vi "SetAttributeViBoolean.vi"(7 "AttributeValue (Off)":bool, 8 "error in (no error)":errorcluster {"code" format="%.0x"}, 9 "AttributeID":u32(ring)=1150179 items=["ACQUISITION_ADC_DITHER_AUTO_ENABLED"=1150179, "ACQUISITION_ADC_DITHER_ENABLED"=1150180, "ACQUISITION_CONTINUOUS_SWEEP_MODE_ENABLED"=1150879, "ANALOGDEMODULATOR_ENABLED"=1150558, "ATTENUATION_AUTO"=1250003, "CALIBRATION_RFPRESELECTOR_AUTO_ALERT_ENABLED"=1150773, "DETECTOR_TYPE_AUTO"=1250005, "DISPLAY_ANNOTATION_ACTIVE_FUNCTION_ENABLED"=1150201, "DISPLAY_ANNOTATION_ENABLED"=1150182, "DISPLAY_ANNOTATION_GRATICULE_ENABLED"=1150189, "DISPLAY_ANNOTATION_MEAS_BAR_ENABLED"=1150200, "DISPLAY_ANNOTATION_SCREEN_ENABLED"=1150202, "DISPLAY_ANNOTATION_TRACE_ENABLED"=1150203, "DISPLAY_ENABLED"=1150117, "DISPLAY_FREQUENCY_LINE_ENABLED"=1150813, "DISPLAY_FULL_SCREEN_ENABLED"=1150118, "DISPLAY_LINE_ENABLED"=1150190, "DISPLAY_MENU_ENABLED"=1150183, "EXTERNAL_MIXER_BIAS_ENABLED"=1250903, "EXTERNAL_MIXER_CONVERSION_LOSS_TABLE_ENABLED"=1250905, "EXTERNAL_MIXER_ENABLED"=1250906, "FREQUENCY_CENTER_STEP_AUTO_ENABLED"=1150544, "FREQUENCY_GLOBAL_CENTER_ENABLED"=1150809, "FREQUENCY_GLOBAL_EXTEND_LOW_BAND_ENABLED"=1150810, "FREQUENCY_SPAN_TO_RESOLUTION_BANDWIDTH_RATIO_AUTO_ENABLED"=1150553, "FREQUENCY_SYNTHESIS_AUTO_ENABLED"=1150545, "INPUT_IF_FFT_IF_GAIN_AUTO_ENABLED"=1150566, "INPUT_IF_SWEPT_IF_GAIN_AUTO_ENABLED"=1150567, "INPUT_RF_AUTO_RANGE_ENABLED"=1150587, "INPUT_RF_CORRECTION_ENABLED"=1150574, "INPUT_RF_CORRECTIONS_ALL_ENABLED"=1150576, "INPUT_RF_CORRECTIONS_NOISE_FLOOR_EXTENSTION_ENABLED"=1150741, "INPUT_RF_PREAMP_ENABLED"=1150573, "INPUT_RF_PRESELECTOR_ENABLED"=1150775], 10 "RepCapIdentifier":string, 11 "instrument handle":refnum<k15>) -> (0 "error out":errorcluster {"code" format="%.0x"}, 3 "instrument handle out":refnum<k15>)   [LabVIEW 2009, in "Keysight XSAn.lvlib"]
doc: "Sets a Boolean attribute from the instrument driver.\nThe following Attributes are supported:\n\nACQUISITION_ADC_DITHER_AUTO_ENABLED\nACQUISITION_ADC_DITHER_ENABLED\nACQUISITION_CONTINUOUS_SWEEP_MODE_ENABLED\nANALOGDEMODULATOR_ENABLED\nATTENUATION_AUTO\nCALIBRATION_RFPRESELECTOR_AUTO_ALERT_ENABLED\nDETECTOR_TYPE_AUTO\nDISPLAY_ANNOTATION_ACTIVE_FUNCTION_ENABLED\nDISPLAY_ANNOTATION_ENABLED\nDISPLAY_ANNOTATION_GRATICULE_ENABLED\nDISPLAY_ANNOTATION_MEAS_BAR_ENABLED\nDISPLAY_ANNOTATION_SCREEN_ENABLED\nDISPLAY_ANNOTATION_TRACE_ENABLED\nDISPLAY_ENABLED\nDISPLAY_FREQUENCY_LINE_ENABLED\nDISPLAY_FULL_SCREEN_ENABLED\nDISPLAY_LINE_ENABLED\nDISPLAY_MENU_ENABLED\nEXTERNAL_MIXER_BIAS_ENABLED\nEXTERNAL_MIXER_CONVERSION_LOSS_TABLE_ENABLED\nEXTERNAL_MIXER_ENABLED\nFREQUENCY_CENTER_STEP_AUTO_ENABLED\nFREQUENCY_GLOBAL_CENTER_ENABLED\nFREQUENCY_GLOBAL_EXTEND_LOW_BAND_ENABLED\nFREQUENCY_SPAN_TO_RESOLUTION_BANDWIDTH_RATIO_AUTO_ENABLED\nFREQUENCY_SYNTHESIS_AUTO_ENABLED\nINPUT_IF_FFT_IF_GAIN_AUTO_ENABLED\nINPUT_IF_SWEPT_IF_GAIN_AUTO_ENABLED\nINPUT_RF_AUTO_RANGE_ENABLED\nINPUT_RF_CORRECTION_ENABLED\nINPUT_RF_CORRECTIONS_ALL_ENABLED\nINPUT_RF_CORRECTIONS_NOISE_FLOOR_EXTENSTION_ENABLED\nINPUT_RF_PREAMP_ENABLED\nINPUT_RF_PRESELECTOR_ENABLED"
uses:
  <instrlib>/Keysight XSAn/Keysight XSAn.lvlib
  AgXSAn.dll
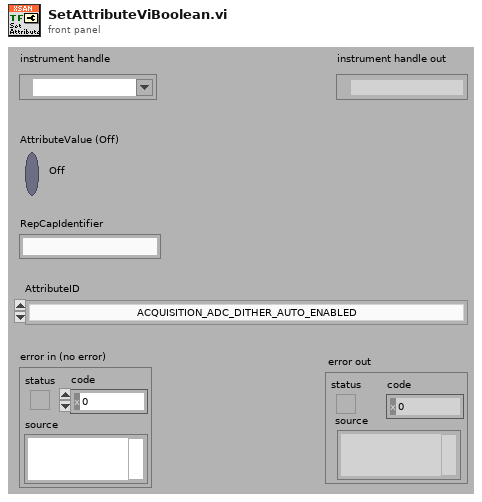
[diagram p1: front panel]
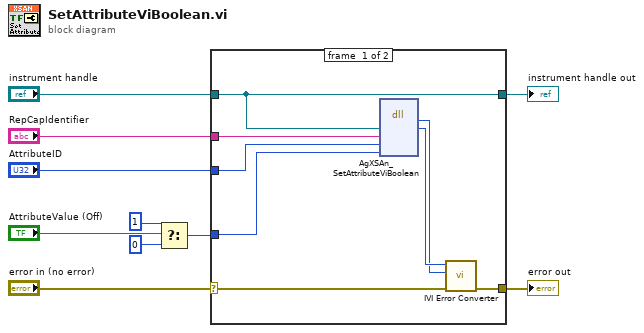
[diagram p0: block diagram]
diagram:
  n1 = Select(t=u16 1, s="AttributeValue (Off)", f=u16 0) -> (s? t:f=w2:u16)
  n2 = case shown="No Error" "error in (no error)" {
    selector: "error in (no error)" -> [w16 w20]
    tunnel: [w15 w20] -> w10
    tunnel: "instrument handle" -> [w11 w19]
    tunnel: "RepCapIdentifier" -> [w14 _]
    tunnel: "AttributeID" -> [w13 _]
    tunnel: w2 -> [w12 _]
    tunnel: [w11 w19] -> w1
    frame #0 {
      n3 = dll-call lib="AgXSAn**.dll" fn="AgXSAn_SetAttributeViBoolean"("Vi"=w11, "RepCapIdentifier"=w14, "AttributeID"=w13, "AttributeValue"=w12) -> ("return type"=w17:i32, "Vi"=w18:u32)  [unwired: 6 in, 2 out]
      n4 = call <instrlib>:"IVI Error Converter.vi"("error in (no error)"=w16, "IVI error code (0)"=w17, "instrument handle"=w18) -> ("error out"=w15:errorcluster)  [unwired: 7 in, 1 out]
    }
    frame #1 {
    }
  }
  "error out" <- w10
  "instrument handle out" <- w1
